vi "SC TCP SoundCheck Control - ready.vi"(8 "error in (no error)":errorcluster, 11 "connection ID in":refnum<k5>) -> (0 "error out":errorcluster, 2 "ready?":bool, 3 "connection ID out":refnum<k5>)   [LabVIEW 2018]
uses:
  <vilib>/Utility/error.llb/Error Cluster From Error Code.vi
  <vilib>/ErrorRing/Error Ring.xnode
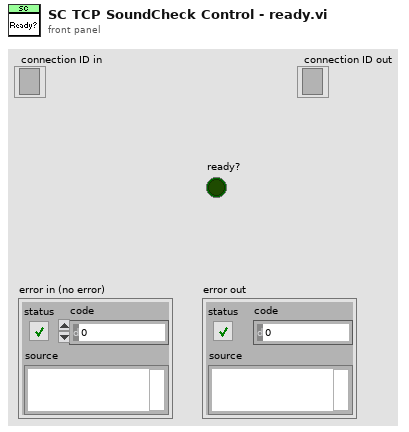
[diagram p1: front panel]
types:
  T1 = typedef "SC TCP SoundCheckStatus.ctl" = cluster{"Busy":bool}
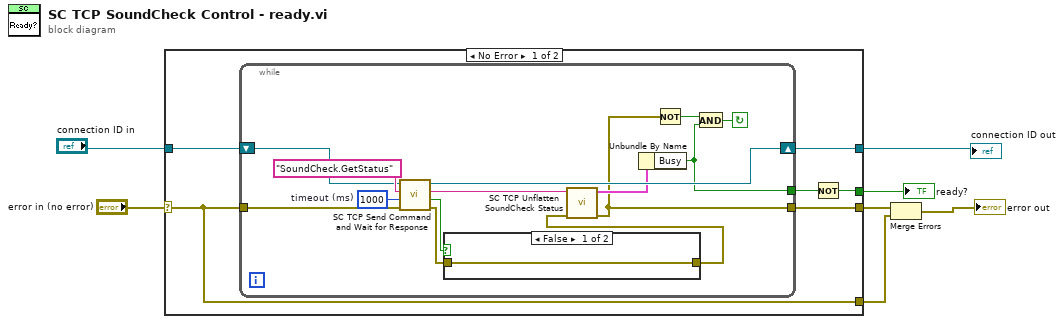
[diagram p0: block diagram]
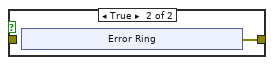
[diagram p2: hidden frame]
diagram:
  n1 = case shown="No Error" "error in (no error)" {
    selector: "error in (no error)" -> [w8 w34]
    tunnel: [w13 w35] -> w3
    tunnel: "connection ID in" -> [w11 w35]
    tunnel: [w12 w34] -> w7
    tunnel: [w9 _] -> w5
    tunnel: [w8 w34] -> w1
    frame No Error {
      n2 = while {
        shift-right: [w27] -> w13
        shift-left: w11 -> [w24]
        tunnel: [w21] -> w10
        tunnel: w8 -> [w17]
        tunnel: [w18] -> w12
        stop <- w20 continue-if-true
        w25 = 1000  # timeout (ms)
        n3 = call "SC TCP Send Command and Wait for Response.vi"("error in (no error)"=w17, "timeout (10000 ms)"=w25, "Command"="SoundCheck.GetStatus", "TCP Network Connection in"=w24) -> ("error out"=w15:errorcluster, "Timed Out"=w16:bool, "Response"=w23:string, "TCP Network Connection out"=w27:refnum<k5>)  [unwired: 4 in]
        n4 = case shown="False" w16 {
          tunnel: w15 -> [w28 _]
          tunnel: [w28 w29] -> w14
          frame False {
          }
          frame True {
            n5 = xnode "Error Ring"() -> ("error out"=w29:errorcluster)
          }
        }
        n6 = call "SC TCP Unflatten SoundCheck Status.vi"("error in"=w14, "Response JSON"=w23) -> ("error out"=w18:errorcluster, "Return"=w22:T1)  [unwired: 8 in]
        n7 = Unbundle By Name(w22) -> ("Busy"=w21:bool)
        n8 = Not(x=w18) -> (.not. x?=w19:bool)
        n9 = And(x=w19, y=w21) -> (x .and. y?=w20:bool)
      }
      n10 = Not(x=w10) -> (.not. x?=w9:bool)
    }
    frame Error {
    }
  }
  "ready?" <- w5
  "connection ID out" <- w3
  n11 = Merge Errors(w7, w1) -> (→"error out":errorcluster)
